vi "Get Oldest.vi"(0 "Tree Reference In":refnum<vi>, 5 "error in (no error)":errorcluster) -> (14 "Tree Reference Out":refnum<vi>, 16 "Oldest Item Tags":string[](array[string]), 19 "error out":errorcluster)   [LabVIEW 2011, in "VITesterUtilities.lvlib"]
doc: "Collects and returns all tags of oldest (leftmost) items in the tree."
uses:
  Libraries/VITesterUtilities.lvlib
panel:
  # "VI INPUTS"
  # "VI OUTPUTS"
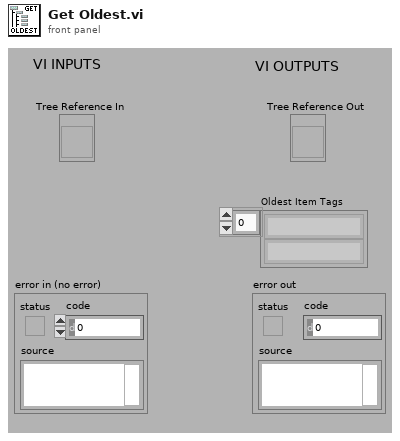
[diagram p1: front panel]
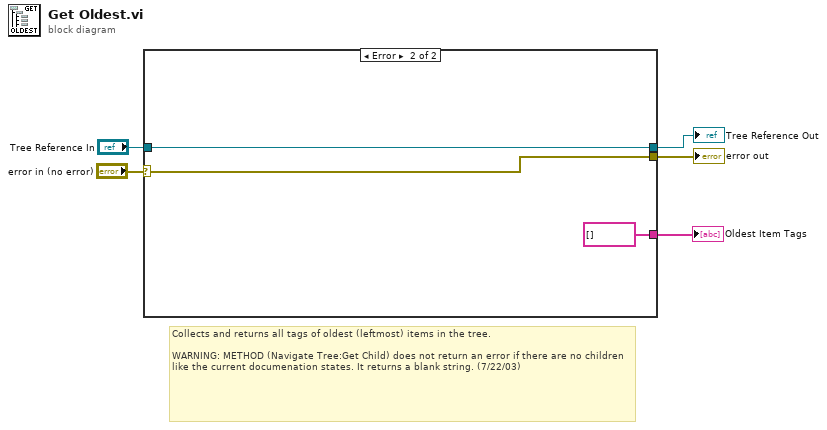
[diagram p0: block diagram]
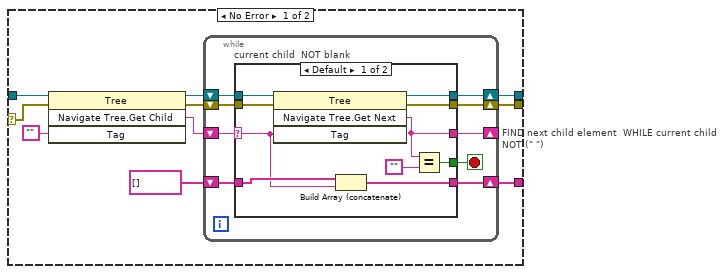
[diagram p2: hidden frame]
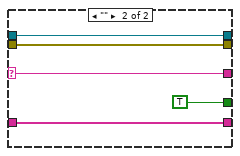
[diagram p3: hidden frame]
diagram:
  # "Collects and returns all tags of oldest (leftmost) items in the tree.\n\nWARNING: METHOD (Navigate Tree:Get Child) does not return an error if there are no children like the current documenation states. It returns a blank string. (7/22/03)"
  n1 = case shown="Error" "error in (no error)" {
    selector: "error in (no error)" -> [w8 w41]
    tunnel: "Tree Reference In" -> [w9 w42]
    tunnel: [w12 w42] -> w4
    tunnel: [w11 string[] []] -> w3
    tunnel: [w10 w41] -> w2
    frame No Error {
      n2 = invoke class="Tree" method="Navigate Tree.Get Child"(reference=w9, error in=w8, "Tag"="") -> (reference out=w14:refnum<vi>, error out=w15:errorcluster, "Navigate Tree:Get Child"=w6:string)  [unwired: 1 in, 1 out]
      n3 = while "FIND next child element  WHILE current child  NOT (\" \")" {
        shift-right: [w22] -> w11
        shift-left: string[] [] -> [w21]
        shift-right: [w23] -> w10
        shift-left: w15 -> [w17]
        shift-right: [w19] -> _
        shift-left: w6 -> [w16]
        shift-right: [w18] -> w12
        shift-left: w14 -> [w24]
        stop <- w20 stop-if-true
        n4 = case "current child  NOT blank" shown="Default" w16 {
          selector: w16 -> [w25 w36]
          tunnel: w24 -> [w34 w38]
          tunnel: [w33 w37] -> w23
          tunnel: [w32 w35] -> w22
          tunnel: w21 -> [w31 w35]
          tunnel: [w28 TRUE] -> w20
          tunnel: [w29 w36] -> w19
          tunnel: [w27 w38] -> w18
          tunnel: w17 -> [w26 w37]
          frame Default {
            n5 = invoke class="Tree" method="Navigate Tree.Get Next"(reference=w34, error in=w26, "Tag"=w25) -> (reference out=w27:refnum<vi>, error out=w33:errorcluster, "Navigate Tree:Get Next Item"=w29:string)  [unwired: 1 in, 1 out]
            n6 = Build Array (concatenate)(w31, w25) -> (w32:string[])
            n7 = Equal?(x=w29, y="") -> (x = y?=w28:bool)
          }
          frame "" {
          }
        }
      }
    }
    frame Error {
    }
  }
  "Oldest Item Tags" <- w3
  "Tree Reference Out" <- w4
  "error out" <- w2
